vi "Limelight Aiming and Range.vi"() -> ()   [LabVIEW 2019]
uses:
  Framework/Robot Global Data.vi
panel:
  in  "KpAim":dbl=-0.1
  in  "KpDistance":dbl=-0.1
  in  "Min Aim Command":dbl=0.05
  in  "tx":dbl
  in  "ty":dbl
  out "Heading Error":dbl
  out "Distance Error":dbl
  out "Steering Adjust":dbl
  out "Distance Adjust":dbl
  in  "Left Command":dbl
  in  "Right Command":dbl
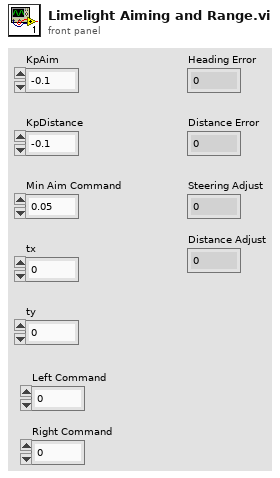
[diagram p1: front panel]
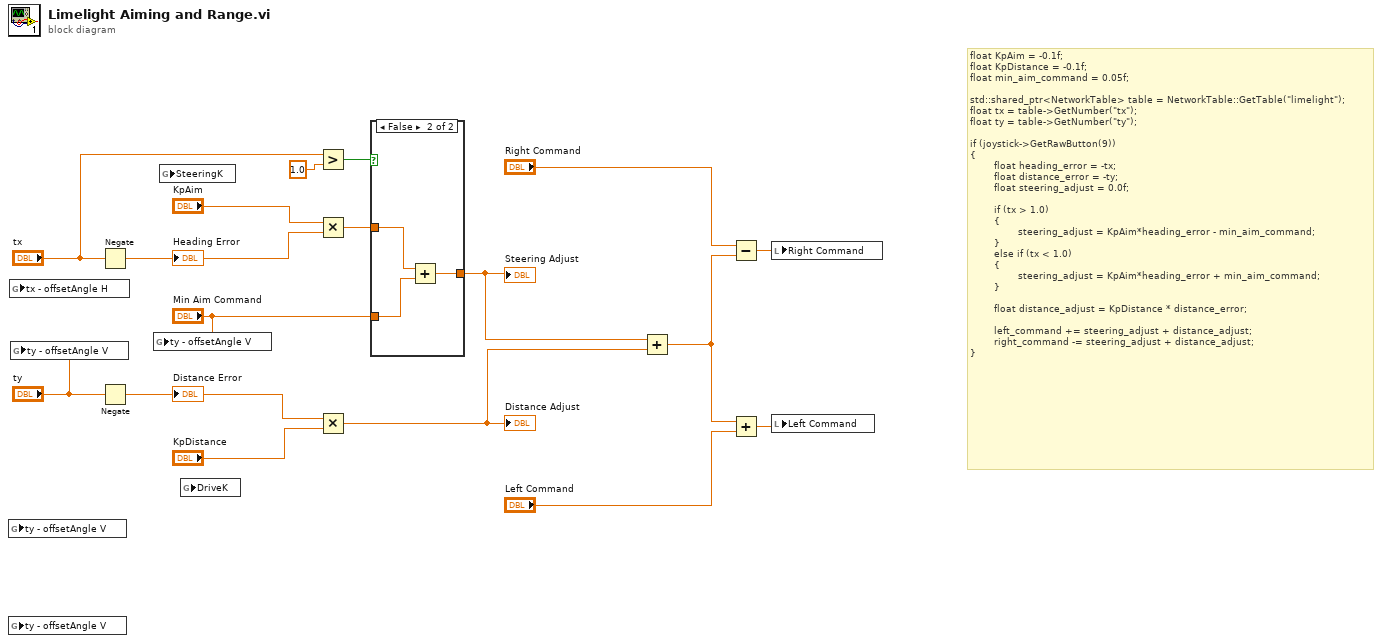
[diagram p0: block diagram]
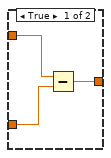
[diagram p2: hidden frame]
diagram:
  # "float KpAim = -0.1f;\nfloat KpDistance = -0.1f;\nfloat min_aim_command = 0.05f;\n\nstd::shared_ptr<NetworkTable> table = NetworkTable::GetTable(\"limelight\");\nfloat tx = table->GetNumber(\"tx\");\nfloat ty = table->GetNumber(\"ty\");\n\nif (joystick->GetRawButton(9))\n{\n        float heading_error = -tx;\n        float distance_error = -ty;\n        float steering_adjust = 0.0f;\n\n        if (tx > 1.0)\n        {\n                steering_adjust = KpAim*heading_error - min_aim_command;\n        }\n        else if (tx < 1.0)\n        {\n                steering_adjust = KpAim*heading_error + min_aim_command;\n        }\n\n        float distance_adjust = KpDistance * distance_error;\n\n        left_command += steering_adjust + distance_adjust;\n        right_command -= steering_adjust + distance_adjust;\n}"
  n1 = global read "Robot Global Data.vi" "ty - offsetAngle V"() -> ()  [unwired: 1 in]
  n2 = global read "Robot Global Data.vi" "ty - offsetAngle V"() -> ()  [unwired: 1 in]
  n3 = global read "Robot Global Data.vi" "tx - offsetAngle H"() -> ()  [unwired: 1 in]
  n4 = global write "Robot Global Data.vi" "ty - offsetAngle V"("ty") -> ()
  n5 = Negate(x="tx") -> (-x=w7:dbl)
  "Heading Error" <- w7
  n6 = Negate(x="ty") -> (-x=w10:dbl)
  "Distance Error" <- w10
  n7 = global write "Robot Global Data.vi" "ty - offsetAngle V"("Min Aim Command") -> ()
  n8 = global read "Robot Global Data.vi" "SteeringK"() -> ()  [unwired: 1 in]
  n9 = global read "Robot Global Data.vi" "DriveK"() -> ()  [unwired: 1 in]
  n10 = Greater?(x="tx", y=1.0) -> (0:w5:bool)
  n11 = Multiply(x="KpAim", y=w7) -> (x*y=w8:dbl)
  n12 = Multiply(x=w10, y="KpDistance") -> (x*y=w12:dbl)
  "Distance Adjust" <- w12
  n13 = case shown="False" w5 {
    tunnel: w8 -> [w20 w23]
    tunnel: "Min Aim Command" -> [w19 w22]
    tunnel: [w18 w21] -> w11
    frame True {
      n14 = Subtract(x=w20, y=w19) -> (x-y=w18:dbl)
    }
    frame False {
      n15 = Add(x=w23, y=w22) -> (x+y=w21:dbl)
    }
  }
  "Steering Adjust" <- w11
  n16 = Add(x=w11, y=w12) -> (x+y=w16:dbl)
  n17 = Subtract(x="Right Command", y=w16) -> (x-y=w17:dbl)
  n18 = Add(x=w16, y="Left Command") -> (x+y=w13:dbl)
  n19 = local write "Right Command"(w17) -> ()
  n20 = local write "Left Command"(w13) -> ()
